vi "subFlexRIO5761.vi"() -> ()   [LabVIEW 2013]
uses:
  <vilib>/eio/EIONode/EIONode.xnode
  <vilib>/Platform/TimedLoop/XDataNode/wakeup.ctl
  <vilib>/Platform/TimedLoop/XDataNode/XDNodeRunTimeDep.lvlib
  <vilib>/Platform/TimedLoop/XDataNode/nitl_modes.ctl
  <vilib>/Platform/TimedLoop/XDataNode/timing_clust.ctl
  <vilib>/Platform/TimedLoop/XDataNode/XDataNode.xnode
  libs/common/GlobalReg.vi
  libs/IRIO.lvlib
  libs/ctl/SelectedChannels.ctl
  libs/FlexRIO/FlexRIO-DMA-DAQ&BUFFERING-5761.vi
  libs/ctl/NumberOfBuffers.ctl
  libs/ctl/NumberOfChannels.ctl
  <vilib>/rvi/eio/common/nirviEmuTemplateMethod_errors.vi
  libs/ctl/DMAConfigParams.ctl
  libs/FlexRIO/FlexRIO-DMA-DAQ-5761.vi
panel:
  in  "Tab Control":T1(tab)=enum."Mandatory Resources"
  out "Platform":enum8{"FlexRIO", "cRIO", "RSeries"}(ring)
  out "FPGAVIversion":u8[](array[numeric])=[1, 1]
  out "Expected IO Module ID":u32 format="%x"
  out "DevProfile":u8 format="%x"
  out "InsertedIOModule ID":u32 format="%x"
  out "DevTemp":i16=-10244
  out "DevQualityStatus":u8=1
  out "InitDone":bool
  out "RIOAdapterCorrect":bool
  in  "DebugMode":bool
  in  "DAQStartStop":bool
  out "Fref":u32=125000000
  out "DMATtoHOSTNCh":u16[](array[numeric])=[4]
  out "DMATtoHOSTFrameType":u8[](array[numeric])
  out "DMATtoHOSTSampleSize":u8[](array[numeric])=[2]
  out "DMATtoHOSTBlockNWords":u16[](array[numeric])=[4096]
  out "DMATtoHOSTOverflows":u16
  in  "DMATtoHOSTEnable0":bool
  in  "DMATtoHOSTSamplingRate0":u16=10000
  in  "SGSignalType0":u8
  in  "AOEnable0":bool
  in  "AOEnable1":bool
  in  "AO1":i32
  in  "SGUpdateRate1":u32=40
  in  "SGFreq1":u32=100000
  in  "SGPhase1":u32
  in  "SGAmp1":u16
  in  "SGSignalType1":u8
  in  "AO0":i32
  in  "SGAmp0":u16
  in  "SGFreq0":u32=100000
  in  "SGPhase0":u32
  in  "SGUpdateRate0":u32=40
  in  "auxDO0":bool
  in  "auxDO1":bool
  in  "auxDO2":bool
  in  "auxDO5":bool
  in  "auxDO4":bool
  in  "auxDO3":bool
  out "auxDI0":bool
  out "auxDI1":bool
  out "auxDI2":bool
  out "auxDI3":bool
  out "auxDI4":bool
  out "auxDI5":bool
  in  "auxAO0":i32
  in  "auxAO1":i32
  in  "auxAO2":i32
  in  "auxAO3":i32
  in  "auxAO4":i32
  in  "auxAO5":i32
  out "auxAI0":i32
  out "auxAI1":i32
  out "auxAI2":i32
  out "auxAI3":i32
  out "auxAI4":i32
  out "auxAI5":i32
  out "SGNo":u8=2 format="%x"
  out "SGFref1":u32=100000000 caption="SGFref0"
  out "SGFref0":u32=100000000
  out "auxAI9":i32
  out "auxAI10":i32
  # "FPGA CONFIGURATION"
  # "0 -> to HOST\n1 -> to GPU"
  # "DEVICE AND MODULE STATUS"
  # "DATA ACQUISITION CONTROL"
  # "DMA CHANNELS CONFIGURATION"
  # "The size of these arrays must match the number of implemented DMA Channels.\n\nThe array item value indicates the corresponding parameter for this DMA Channel"
  # "Number of channels"
  # "Frame  Type:   0 -> Format A\n                      1 -> Format B"
  # "Sample Size:    1 Byte    2 Bytes, \n                      4 Bytes   8 Bytes"
  # "Block Length"
  # "DMA CHANNELS STATUS"
  # "DMA 0"
  # "DMA 1"
  # "DMA 2"
  # "Inputs"
  # "Aux \nDigital Inputs"
  # "Aux \nAnalog Inputs"
  # "Digital Inputs"
  # "Outputs"
  # "Number of WF gen"
  # "Analog Outputs"
  # "Aux Digital \nOutput"
  # "Digital\nOutputs"
  # "Aux Analog \nOutput"
  # "Signal Generator 1"
  # "Signal Generator 0"
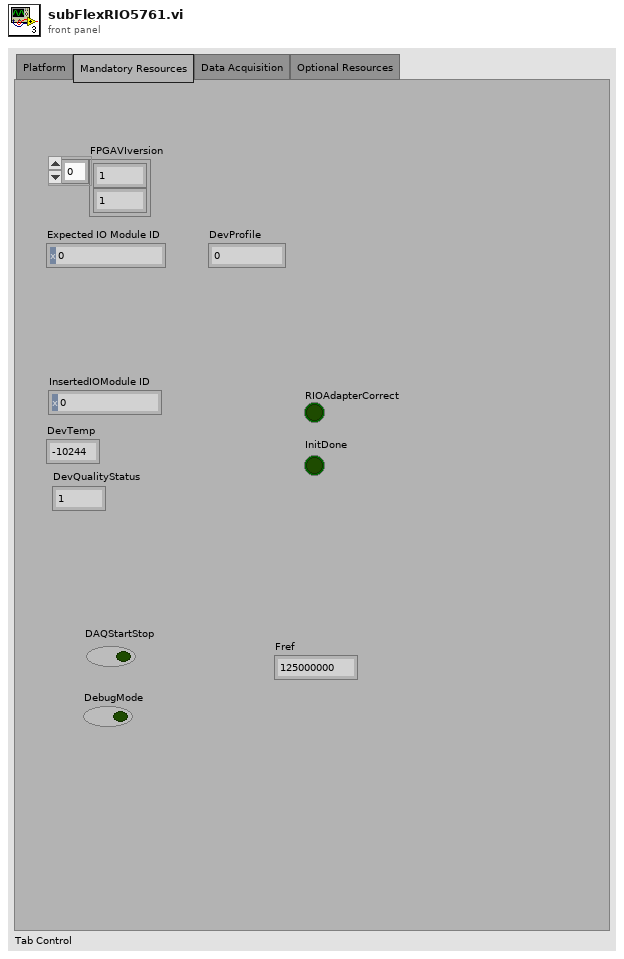
[diagram p1: front panel]
types:
  T1 = enum32{"Platform", "Mandatory Resources", "Data Acquisition", "Optional Resources"}
  T2 = typedef "IRIO.lvlib/DMAConfigParams.ctl" = u16
  T3 = cluster{"DMATtoHOSTNCh":T2[], "DMATtoHOSTFrameType":u8[], "DMATtoHOSTSampleSize":u8[], "DMATtoHOSTBlockNWords":u16[]}
  T4 = cluster{"CH0BUFFER":refnum<k21>, "CH1BUFFER":refnum<k21>, "CH2BUFFER":refnum<k21>, "CH3BUFFER":refnum<k21>, "CH0DMANumber ":i32, "CH1DMANumber":i32, "CH2DMANumber":i32, "CH3DMANumber":i32}
  T5 = cluster{"Expected IO Module ID":u32, "InsertedIOModule ID":u32, "RIOAdapterCorrect":bool}
  T6 = typedef "XDNodeRunTimeDep.lvlib/timing_clust.ctl" = cluster{"Expected End [f-1]":u64, "Actual End [f-1]":u64, "Finished Late? [f-1]":bool, "Expected End [i-1]":u64, "Actual End [i-1]":u64, "Finished Late? [i-1]":bool, "Expected Start [i]":u64, "Actual Start [i]":u64, "Expected Start [f]":u64, "Actual Start [f]":u64, "Source Name":string, "Structure Name":string, "Period":i64, "Deadline":i64, "Offset":i64, "Start":i64, "Priority":i32, "Timeout":i32, "Mode":T7, "Wakeup Reason":T8, "Error":errorcluster, "Source Type":string, "Secondary Source Type":string, "Global End Time":u64, "Global Start Time":u64, "Frame Duration":u64, "Iteration Duration":u64, "Assigned CPU":i32, "I/O Scan Engine Mode":u32}
  T7 = typedef "XDNodeRunTimeDep.lvlib/nitl_modes.ctl" = enum32{"No Change", "Process missed periods, maintain original phase", "Discard missed periods, maintain original phase", "Process missed periods, ignore original phase", "Discard missed periods, ignore original phase"}
  T8 = typedef "XDNodeRunTimeDep.lvlib/wakeup.ctl" = enum32{"Normal", "Aborted", "Asynchronous wakeup", "Timing source error", "Timed loop error", "Timeout"}
  T9 = typedef "IRIO.lvlib/NumberOfBuffers.ctl" = enum16{"0 Buffers", "1 Buffers", "2 Buffers", "3 Buffers", "4 Buffers", "5 Buffers", "6 Buffers", "7 Buffers", "8 Buffers", "9 Buffers", "10 Buffers", "11 Buffers", "12 Buffers"}
  T10 = typedef "IRIO.lvlib/SelectedChannels.ctl" = enum16{"Empty", "AI0", "AI1", "AI2", "AI3", "SignalGenerator0", "SignalGenerator1", "DDCA_PORT0", "DDCA_PORT1", "DDCA_PORT2", "DDCB_PORT0", "DDCB_PORT1", "DDCB_PORT2"}
  T11 = cluster{"CH0BUFFER":refnum<k21>, "CH1BUFFER":refnum<k21>, "CH2BUFFER":refnum<k21>, "CH3BUFFER":refnum<k21>}
  T12 = typedef "IRIO.lvlib/NumberOfChannels.ctl" = enum16{"0 Channels", "1 Channels", "2 Channels", "3 Channels", "4 Channels", "5 Channels", "6 Channels", "7 Channels", "8 Channels", "9 Channels", "10 Channels", "11 Channels", "12 Channels"}
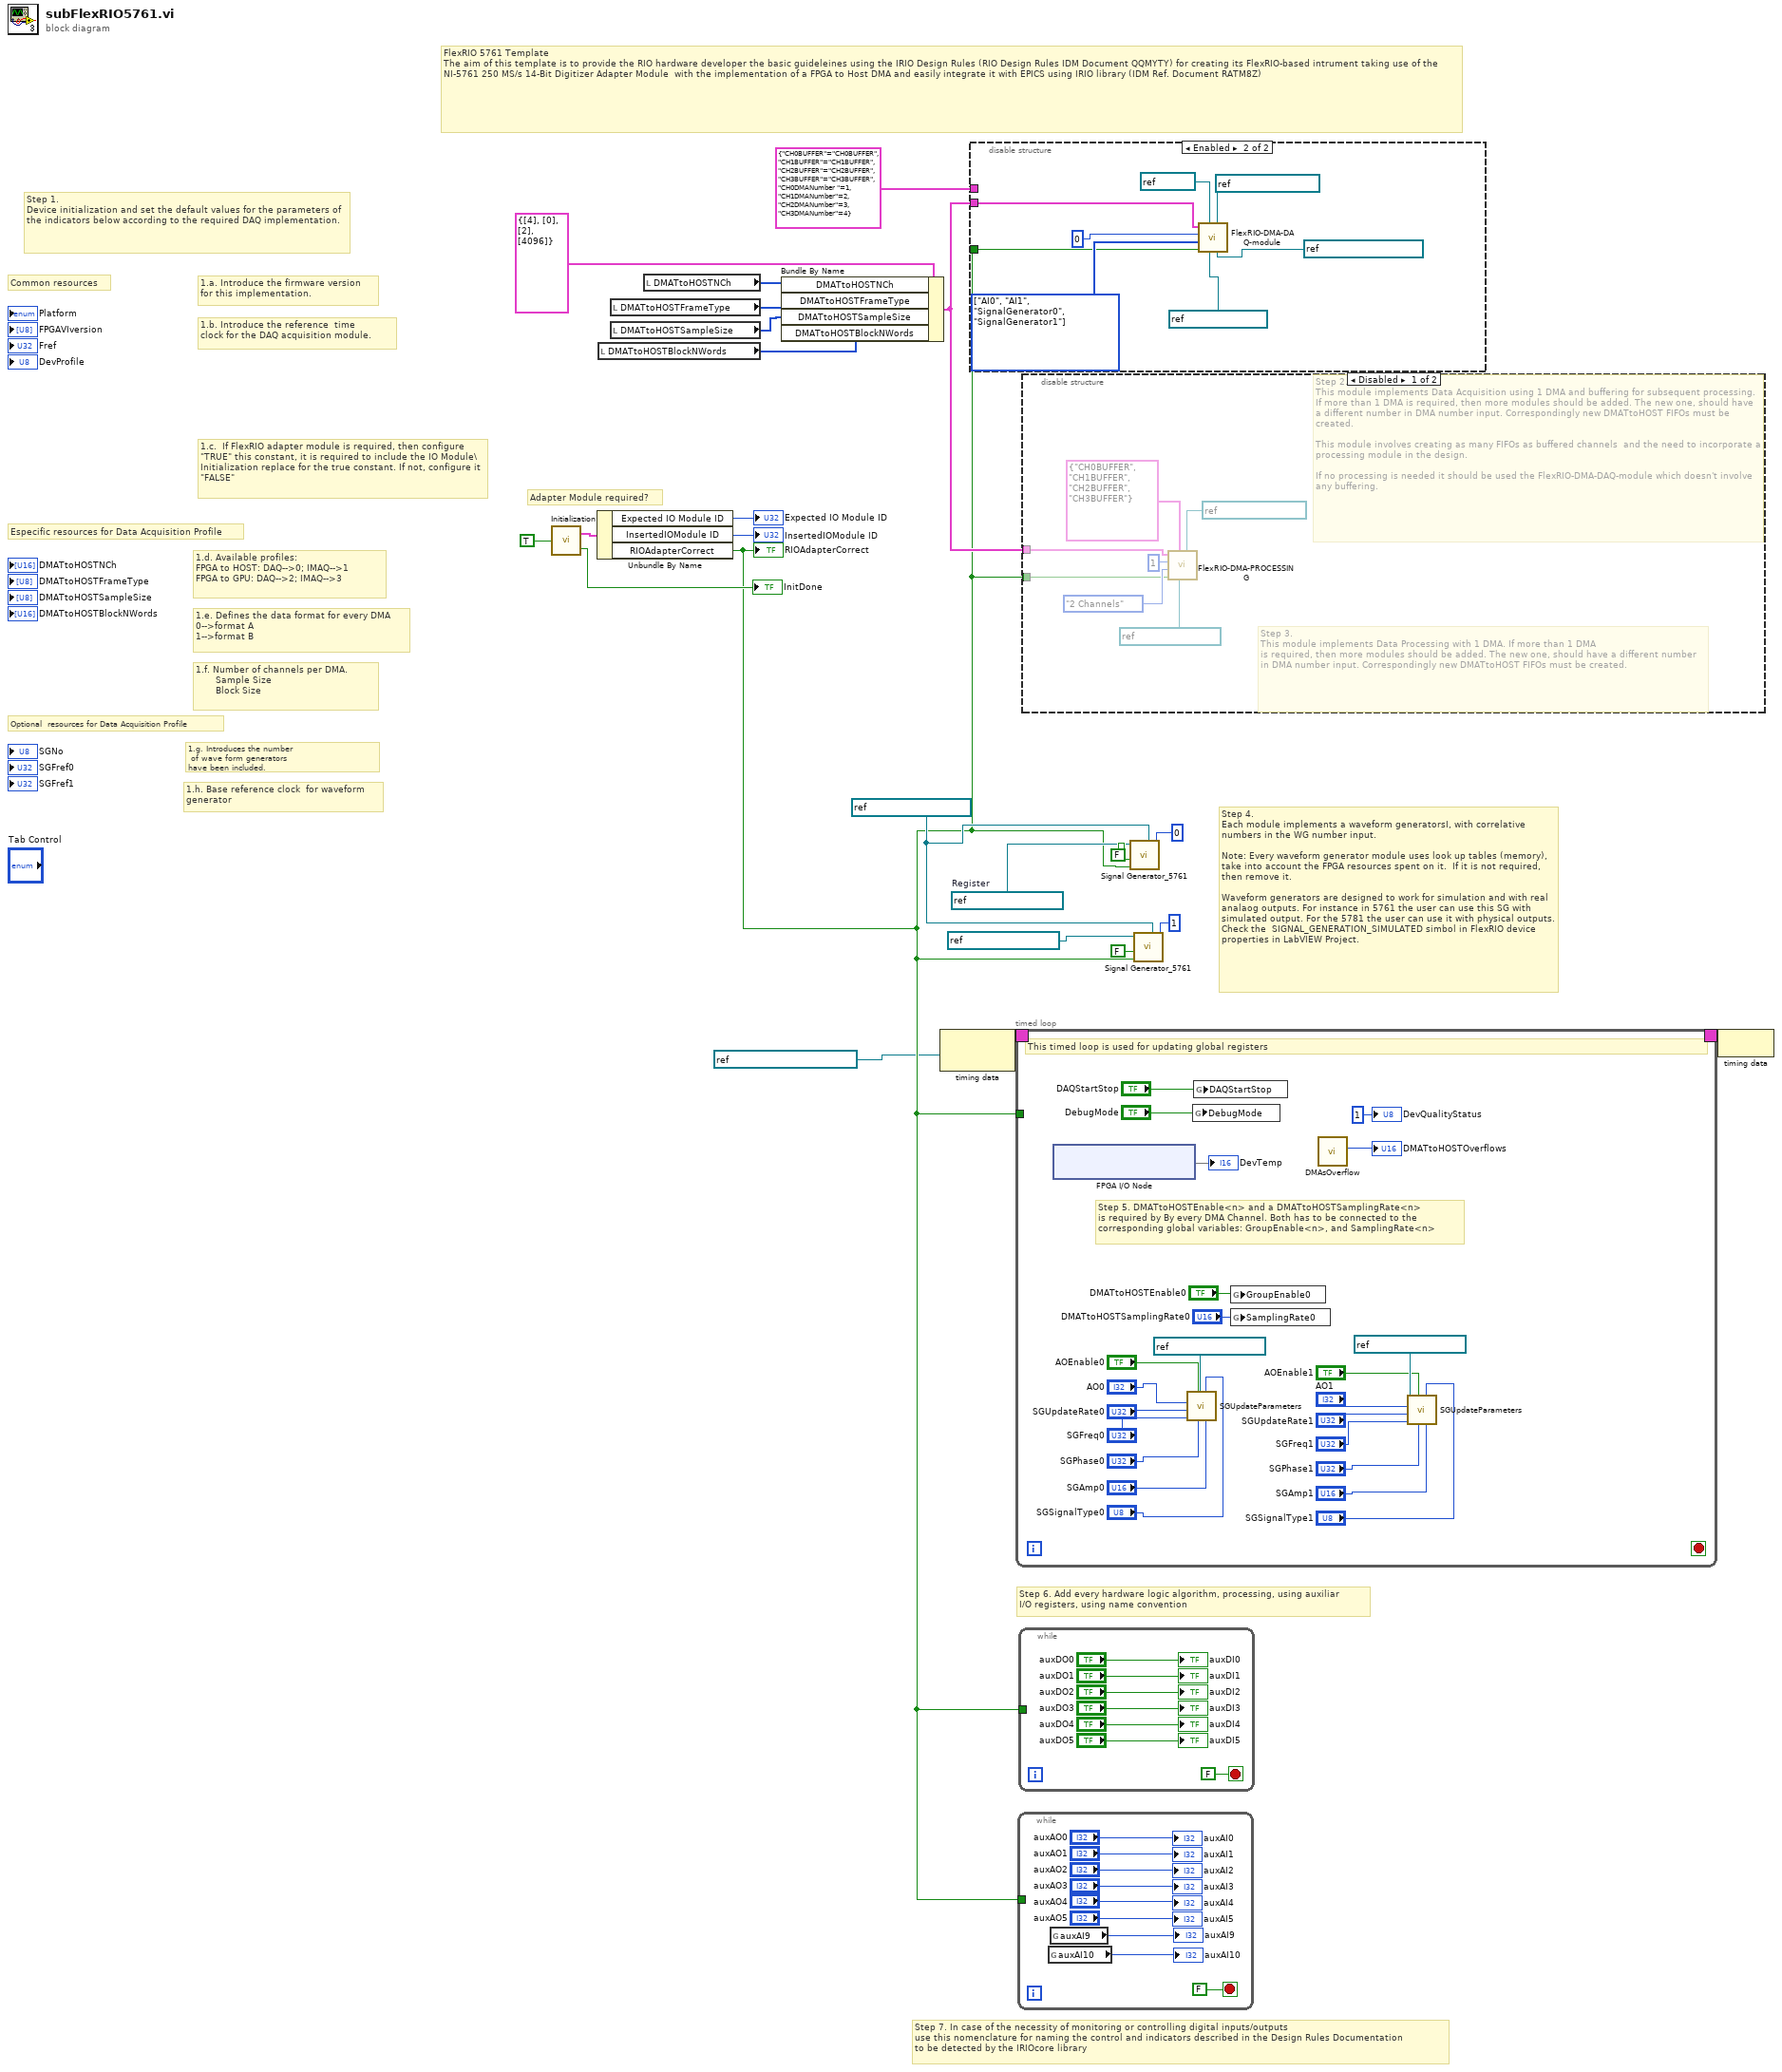
[diagram p0: block diagram]
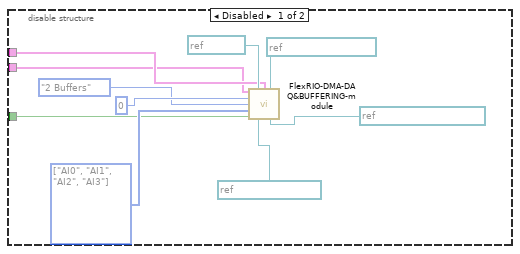
[diagram p2: hidden frame]
diagram:
  w11 = refnum<k21> "SignalGenerator0"  # Register
  w10 = refnum<k21> "IO Module Clock 1" ("Clock in")
  # "Adapter Module required?"
  # "1.h. Base reference clock  for waveform\ngenerator"
  # "1.e. Defines the data format for every DMA\n0-->format A\n1-->format B"
  # "1.c.  If FlexRIO adapter module is required, then configure \"TRUE\" this constant, it is required to include the IO Module\\Initialization replace for the true constant. If not, configure it \"FALSE\""
  # "1.a. Introduce the firmware version \nfor this implementation."
  # "1.b. Introduce the reference  time \nclock for the DAQ acquisition module."
  # "1.g. Introduces the number \n of wave form generators \nhave been included."
  # "1.f. Number of channels per DMA.\n       Sample Size\n       Block Size"
  # "1.d. Available profiles: \nFPGA to HOST: DAQ-->0; IMAQ-->1\nFPGA to GPU: DAQ-->2; IMAQ-->3"
  # "Optional  resources for Data Acquisition Profile"
  # "Especific resources for Data Acquisition Profile"
  # "Common resources"
  # "FlexRIO 5761 Template\nThe aim of this template is to provide the RIO hardware developer the basic guideleines using the IRIO Design Rules (RIO Design Rules IDM Document QQMYTY) for creating its FlexRIO-based intrument taking use of the NI-5761 250 MS/s 14-Bit Digitizer Adapter Module  with the implementation of a FPGA to Host DMA and easily integrate it with EPICS using IRIO library (IDM Ref. Document RATM8Z)"
  # "Step 4.\nEach module implements a waveform generatorsI, with correlative numbers in the WG number input.\n \nNote: Every waveform generator module uses look up tables (memory), take into account the FPGA resources spent on it.  If it is not required, then remove it.\n\nWaveform generators are designed to work for simulation and with real analaog outputs. For instance in 5761 the user can use this SG with simulated output. For the 5781 the user can use it with physical outputs. \nCheck the  SIGNAL_GENERATION_SIMULATED simbol in FlexRIO device properties in LabVIEW Project."
  # "Step 7. In case of the necessity of monitoring or controlling digital inputs/outputs \nuse this nomenclature for naming the control and indicators described in the Design Rules Documentation\nto be detected by the IRIOcore library"
  # "Step 6. Add every hardware logic algorithm, processing, using auxiliar \nI/O registers, using name convention"
  # "Step 1. \nDevice initialization and set the default values for the parameters of the indicators below according to the required DAQ implementation."
  n1 = call "Initialization.vi"("AdapterModuleRequired"=TRUE) -> ("InitDone"=→"InitDone":bool, "IO Module ID"=w20:T5)  [unwired: 2 in]
  n2 = Unbundle By Name(w20) -> ("Expected IO Module ID"=→"Expected IO Module ID":u32, "InsertedIOModule ID"=→"InsertedIOModule ID":u32, "RIOAdapterCorrect"=w3:bool)
  "RIOAdapterCorrect" <- w3
  n3 = local read "DMATtoHOSTBlockNWords"() -> (w14:u16[])
  n4 = local read "DMATtoHOSTFrameType"() -> (w16:u8[])
  n5 = local read "DMATtoHOSTSampleSize"() -> (w15:u8[])
  n6 = local read "DMATtoHOSTNCh"() -> (w17:u16[])
  n7 = Bundle By Name(cluster=T3 {"DMATtoHOSTNCh"=[4], "DMATtoHOSTFrameType"=[0], "DMATtoHOSTSampleSize"=[2], "DMATtoHOSTBlockNWords"=[4096]} ("DMA Control"), "DMATtoHOSTNCh"=w17, "DMATtoHOSTFrameType"=w16, "DMATtoHOSTSampleSize"=w15, "DMATtoHOSTBlockNWords"=w14) -> (w4:T3)
  n8 = node-c288(refnum<k21> "40 MHz Onboard Clock" ("Source Name")) -> (w23:T6)
  n9 = disable-structure shown="Enabled" {
    disable-tunnel: T4 {"CH0BUFFER"="CH0BUFFER", "CH1BUFFER"="CH1BUFFER", "CH2BUFFER"="CH2BUFFER", "CH3BUFFER"="CH3BUFFER", "CH0DMANumber "=1, "CH1DMANumber"=2, "CH2DMANumber"=3, "CH3DMANumber"=4} ("BUFFERS Info") -> [w27 _]
    disable-tunnel: w4 -> [w25 w35]
    disable-tunnel: w3 -> [w24 w34]
    frame Disabled {
      w30 = T10[] [enum."AI0", enum."AI1", enum."AI2", enum."AI3"] items=["Empty", "AI0", "AI1", "AI2", "AI3", "SignalGenerator0", "SignalGenerator1", "DDCA_PORT0", "DDCA_PORT1", "DDCA_PORT2", "DDCB_PORT0", "DDCB_PORT1", "DDCB_PORT2"] ("Selected Channels")
      n10 = call-poly "FlexRIO-DMA-DAQ&BUFFERING-module.vi"("DMA Control"=w25, "IntermediateFIFO"=refnum<k21> "FIFO0", "BUFFERS Info"=w27, "DMATtoHOSTFIFO"=refnum<k21> "DMATtoHOST0", "DMA number"=0, "NumberOfBuffers"=NumberOfBuffers."2 Buffers", "Selected Channels"=w30, "Enable"=w24, "Base Clock"=refnum<k21> "125MHz Clock", "Module Clock"=refnum<k21> "IO Module Clock 0") -> ()  [unwired: 6 in]
    }
    frame Enabled {
      w38 = T10[] [enum."AI0", enum."AI1", enum."SignalGenerator0", enum."SignalGenerator1"] items=["Empty", "AI0", "AI1", "AI2", "AI3", "SignalGenerator0", "SignalGenerator1", "DDCA_PORT0", "DDCA_PORT1", "DDCA_PORT2", "DDCB_PORT0", "DDCB_PORT1", "DDCB_PORT2"] ("Selected Channels")
      n11 = call-poly "FlexRIO-DMA-DAQ-module.vi"("Module Clock"=refnum<k21> "IO Module Clock 0", "DMATtoHOSTFIFO"=refnum<k21> "DMATtoHOST0", "Base Clock"=refnum<k21> "125MHz Clock", "IntermediateFIFO"=refnum<k21> "FIFO0", "Enable"=w34, "Selected Channels"=w38, "DMA number"=0, "DMA Control"=w35) -> ()  [unwired: 4 in]
    }
  }
  n12 = timed-loop {
    timing: w23 -> [_]
    timing-out: [_] -> w22
    tunnel: w3 -> [_]
    stop <- _ stop-if-true
    # "Step 5. DMATtoHOSTEnable<n> and a DMATtoHOSTSamplingRate<n> \nis required by By every DMA Channel. Both has to be connected to the \ncorresponding global variables: GroupEnable<n>, and SamplingRate<n>"
    # "This timed loop is used for updating global registers"
    n13 = xnode "FPGA I/O Node"() -> ("Device Temperature"=→"DevTemp")  [unwired: 1 in, 1 out]
    n14 = call "SGUpdateParameters.vi"("SGAmp0"="SGAmp0", "SGSignalType0"="SGSignalType0", "SGPhase0"="SGPhase0", "AOEnable0"="AOEnable0", "SGFreq0"="SGFreq0", "SGUpdateRate0"="SGUpdateRate0", "AO0"="AO0", "Refnum in"=refnum<k21> "SignalGenerator0") -> ()  [unwired: 3 in, 1 out]
    n15 = global write "GlobalReg.vi" "DebugMode"("DebugMode") -> ()
    n16 = global write "GlobalReg.vi" "DAQStartStop"("DAQStartStop") -> ()
    n17 = global write "GlobalReg.vi" "GroupEnable0"("DMATtoHOSTEnable0") -> ()
    n18 = global write "GlobalReg.vi" "SamplingRate0"("DMATtoHOSTSamplingRate0") -> ()
    n19 = call "DMAsOverflow.vi"() -> ("DMAsOverFlow"=→"DMATtoHOSTOverflows":u16)  [unwired: 11 in]
    n20 = call "SGUpdateParameters.vi"("SGAmp0"="SGAmp1", "SGSignalType0"="SGSignalType1", "SGPhase0"="SGPhase1", "AOEnable0"="AOEnable1", "SGFreq0"="SGFreq1", "SGUpdateRate0"="SGUpdateRate1", "AO0"="AO1", "Refnum in"=refnum<k21> "SignalGenerator1") -> ()  [unwired: 3 in, 1 out]
    "DevQualityStatus" <- u8 1 ("DevQualityStatus")
  }
  n21 = while {
    tunnel: w3 -> [_]
    stop <- FALSE stop-if-true
    n22 = global read "GlobalReg.vi" "auxAI10"() -> (→"auxAI10":i32)
    n23 = global read "GlobalReg.vi" "auxAI9"() -> (→"auxAI9":i32)
    "auxAI0" <- "auxAO0"
    "auxAI1" <- "auxAO1"
    "auxAI2" <- "auxAO2"
    "auxAI3" <- "auxAO3"
    "auxAI4" <- "auxAO4"
    "auxAI5" <- "auxAO5"
  }
  n24 = while {
    tunnel: w3 -> [_]
    stop <- FALSE stop-if-true
    "auxDI0" <- "auxDO0"
    "auxDI1" <- "auxDO1"
    "auxDI2" <- "auxDO2"
    "auxDI3" <- "auxDO3"
    "auxDI4" <- "auxDO4"
    "auxDI5" <- "auxDO5"
  }
  n25 = disable-structure shown="Disabled" {
    disable-tunnel: w4 -> [w87 _]
    disable-tunnel: w3 -> [w84 _]
    frame Disabled {
      # "Step 3.\nThis module implements Data Processing with 1 DMA. If more than 1 DMA \nis required, then more modules should be added. The new one, should have a different number in DMA number input. Correspondingly new DMATtoHOST FIFOs must be created."
      # "Step 2.\nThis module implements Data Acquisition using 1 DMA and buffering for subsequent processing. If more than 1 DMA is required, then more modules should be added. The new one, should have a different number in DMA number input. Correspondingly new DMATtoHOST FIFOs must be created. \n\nThis module involves creating as many FIFOs as buffered channels  and the need to incorporate a processing module in the design.\n\nIf no processing is needed it should be used the FlexRIO-DMA-DAQ-module which doesn't involve any buffering."
      n26 = call "FlexRIO-DMA-PROCESSING.vi"("DMATtoHOSTFIFO"=refnum<k21> "DMATtoHOST1", "Base Clock"=refnum<k21> "100 MHz Clock", "CHBUFFERS"=T11 {"CH0BUFFER"="CH0BUFFER", "CH1BUFFER"="CH1BUFFER", "CH2BUFFER"="CH2BUFFER", "CH3BUFFER"="CH3BUFFER"}, "Enable"=w84, "NumberOfChannels"=NumberOfChannels."2 Channels", "DMA number"=1, "DMA Control"=w87) -> ()  [unwired: 5 in]
    }
    frame Enabled {
    }
  }
  n27 = call "Signal Generator_5761.vi"("Register"=w11, "Drive?"=FALSE, "Enabled"=w3, "Clock in"=w10, "SGNumber"=i16 0) -> ()  [unwired: 4 in]
  n28 = call "Signal Generator_5761.vi"("Register"=refnum<k21> "SignalGenerator1" ("Refnum in"), "Drive?"=FALSE, "Enabled"=w3, "Clock in"=w10, "SGNumber"=i16 1) -> ()  [unwired: 4 in]
  n29 = node-c288(w22) -> ()
